vi "IFwTest.vi"() -> ()   [LabVIEW 2017]
uses:
  <vilib>/Platform/TimedLoop/XDataNode/timing_clust.ctl
  <vilib>/Platform/TimedLoop/XDataNode/nitl_modes.ctl
  <vilib>/Platform/TimedLoop/XDataNode/wakeup.ctl
  <instrlib>/_niInstr/Instruction Framework/v1/FPGA/Helper Classes/Single Address Space Collection/Single Address Space Collection.lvclass
  C:/Program Files (x86)/National Instruments/LabVIEW 2017/instr.lib/_niInstr/Instruction Framework/v1/FPGA/Interfaces/Address Space Collection/Address Space Collection.lvclass
  <instrlib>/_niInstr/FIFO Register Bus/v1/FPGA/niInstr FIFO Register Bus v1 FPGA.lvclass
  C:/Program Files (x86)/National Instruments/LabVIEW 2017/instr.lib/_niInstr/Instruction Framework/v1/FPGA/Interfaces/Instruction Producer/Instruction Producer.lvclass
  <vilib>/rvi/Emulation/niFpgaGetClockAttributes.vi
  <vilib>/rvi/Emulation/niFpgaSctlEmulationGetInTimedLoop.vi
  <vilib>/rvi/Emulation/niFpgaEmulationReportErrorSimple.vi
  <vilib>/rvi/Emulation/niFpgaCriticalErrorInLSC.vi
  <vilib>/rvi/DataTransferAndStorage/Container/Common/niFpgaContainerExecOnDevCompGetState.vi
  <vilib>/rvi/Emulation/niFpgaEmulationIsFPGAContextNoSignature.vi
  <vilib>/rvi/DataTransferAndStorage/Container/Common/niFpgaContainerGetUniqueNameForEmu.vi
  <vilib>/rvi/Memory/Memory_Emulation/niFpgaMemoryEmulationCacheClearOnFirstRun.vi
  <vilib>/rvi/Memory/Memory_Emulation/nirvimemoryEmulationManagerCache_MakeExclusive.vi
  <vilib>/rvi/Memory/Memory_Emulation/niFpgaMemoryEmulationValidateCache.vi
  <vilib>/rvi/Memory/Memory_Emulation/nirvimemoryEmulationManagerCache_InsertValue.vi
  <vilib>/Utility/error.llb/Clear Errors.vi
  <vilib>/rvi/Memory/Memory_Emulation/nirvimemoryEmulationManagerCache_ReleaseExclusive.vi
  <vilib>/rvi/Memory/Memory_Emulation/nirvimemoryEmulationManagerCache_GetValue.vi
  <vilib>/rvi/Memory/Memory_Emulation/nirvimemoryEmulationManagerCache_SetValue.vi
  <vilib>/rvi/Emulation/niFpgaProcessEmulError.vi
  <vilib>/Platform/TimedLoop/XDataNode/XDataNode.xnode
  <vilib>/rvi/DataTransferAndStorage/Container/XNode/niFpgaContainer.xnode
  <vilib>/rvi/DataTransferAndStorage/Register/Emulation/niFpgaRegisterEmulationRefIn.vi
  <instrlib>/_niInstr/Instruction Framework/v1/FPGA/Top Level Bus/Register Configuration/Register Configuration.lvclass
  <vilib>/Platform/TimedLoop/XDataNode/XDNodeRunTimeDep.lvlib
  AddressSpace.lvclass
panel:
  out "numOfInterleaves 2":u8
  out "rampRate 2":sgl
  out "manualInput 2":sgl
  out "perturbAmp 2":sgl
  out "perturbAngleInc 2":fxp<+/-,16,0>
  out "reset 2":bool
  out "state 2":T1(ring)
  out "gains 2":T2
  out "numInterleaves 2":u8
  out "enable 2":bool
  out "triangleInc 2":fxp<+,18,0>
  out "deadband 2":u16
  out "deadband":u16
  out "triangleInc":fxp<+,18,0>
  out "enable":bool
  out "numInterleaves":u8
  out "gains":T2
  out "state":T1(ring)
  out "reset":bool
  out "perturbAngleInc":fxp<+/-,16,0>
  out "perturbAmp":sgl
  out "manualInput":sgl
  out "rampRate":sgl
  out "numOfInterleaves":u8
  in  "fifo reg bus ctrl 0":u32
  out "fifo reg bus status 0":u32
  out "fifo reg bus data 0":u64
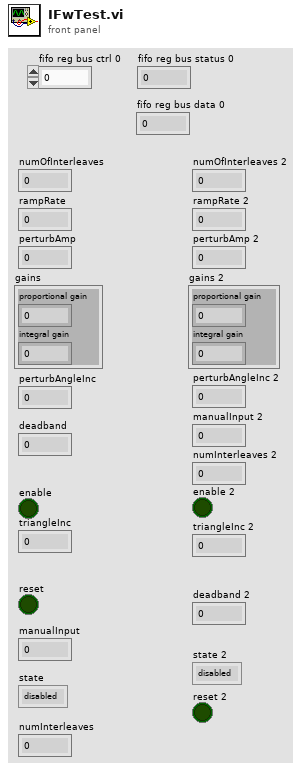
[diagram p1: front panel]
types:
  T1 = enum16{"disabled", "manual", "normal", "perturb"}
  T2 = cluster{"proportional gain":sgl, "integral gain":sgl}
  T3 = typedef "XDNodeRunTimeDep.lvlib/timing_clust.ctl" = cluster{"Expected End [f-1]":u64, "Actual End [f-1]":u64, "Finished Late? [f-1]":bool, "Expected End [i-1]":u64, "Actual End [i-1]":u64, "Finished Late? [i-1]":bool, "Expected Start [i]":u64, "Actual Start [i]":u64, "Expected Start [f]":u64, "Actual Start [f]":u64, "Source Name":string, "Structure Name":string, "Period":i64, "Deadline":i64, "Offset":i64, "Start":i64, "Priority":i32, "Timeout":i32, "Mode":T4, "Wakeup Reason":T5, "Error":errorcluster, "Source Type":string, "Secondary Source Type":string, "Global End Time":u64, "Global Start Time":u64, "Frame Duration":u64, "Iteration Duration":u64, "Assigned CPU":i32, "I/O Scan Engine Mode":u32}
  T4 = typedef "XDNodeRunTimeDep.lvlib/nitl_modes.ctl" = enum32{"No Change", "Process missed periods, maintain original phase", "Discard missed periods, maintain original phase", "Process missed periods, ignore original phase", "Discard missed periods, ignore original phase"}
  T5 = typedef "XDNodeRunTimeDep.lvlib/wakeup.ctl" = enum32{"Normal", "Aborted", "Asynchronous wakeup", "Timing source error", "Timed loop error", "Timeout"}
  T6 = typedef "BuckBoost.lvlib/contSettings.ctl" = cluster{"numberOfInterleaves":refnum<k21>, "rampRate":refnum<k21>, "manualInput":refnum<k21>, "perturbAmp":refnum<k21>, "perturbAngleInc":refnum<k21>, "reset":refnum<k21>, "state":refnum<k21>, "gains":refnum<k21>}
  T7 = typedef "BuckBoost.lvlib/modRegisters.ctl" = cluster{"numberOfInterleaves":refnum<k21>, "Enable":refnum<k21>, "triangleInc":refnum<k21>, "Deadband":refnum<k21>}
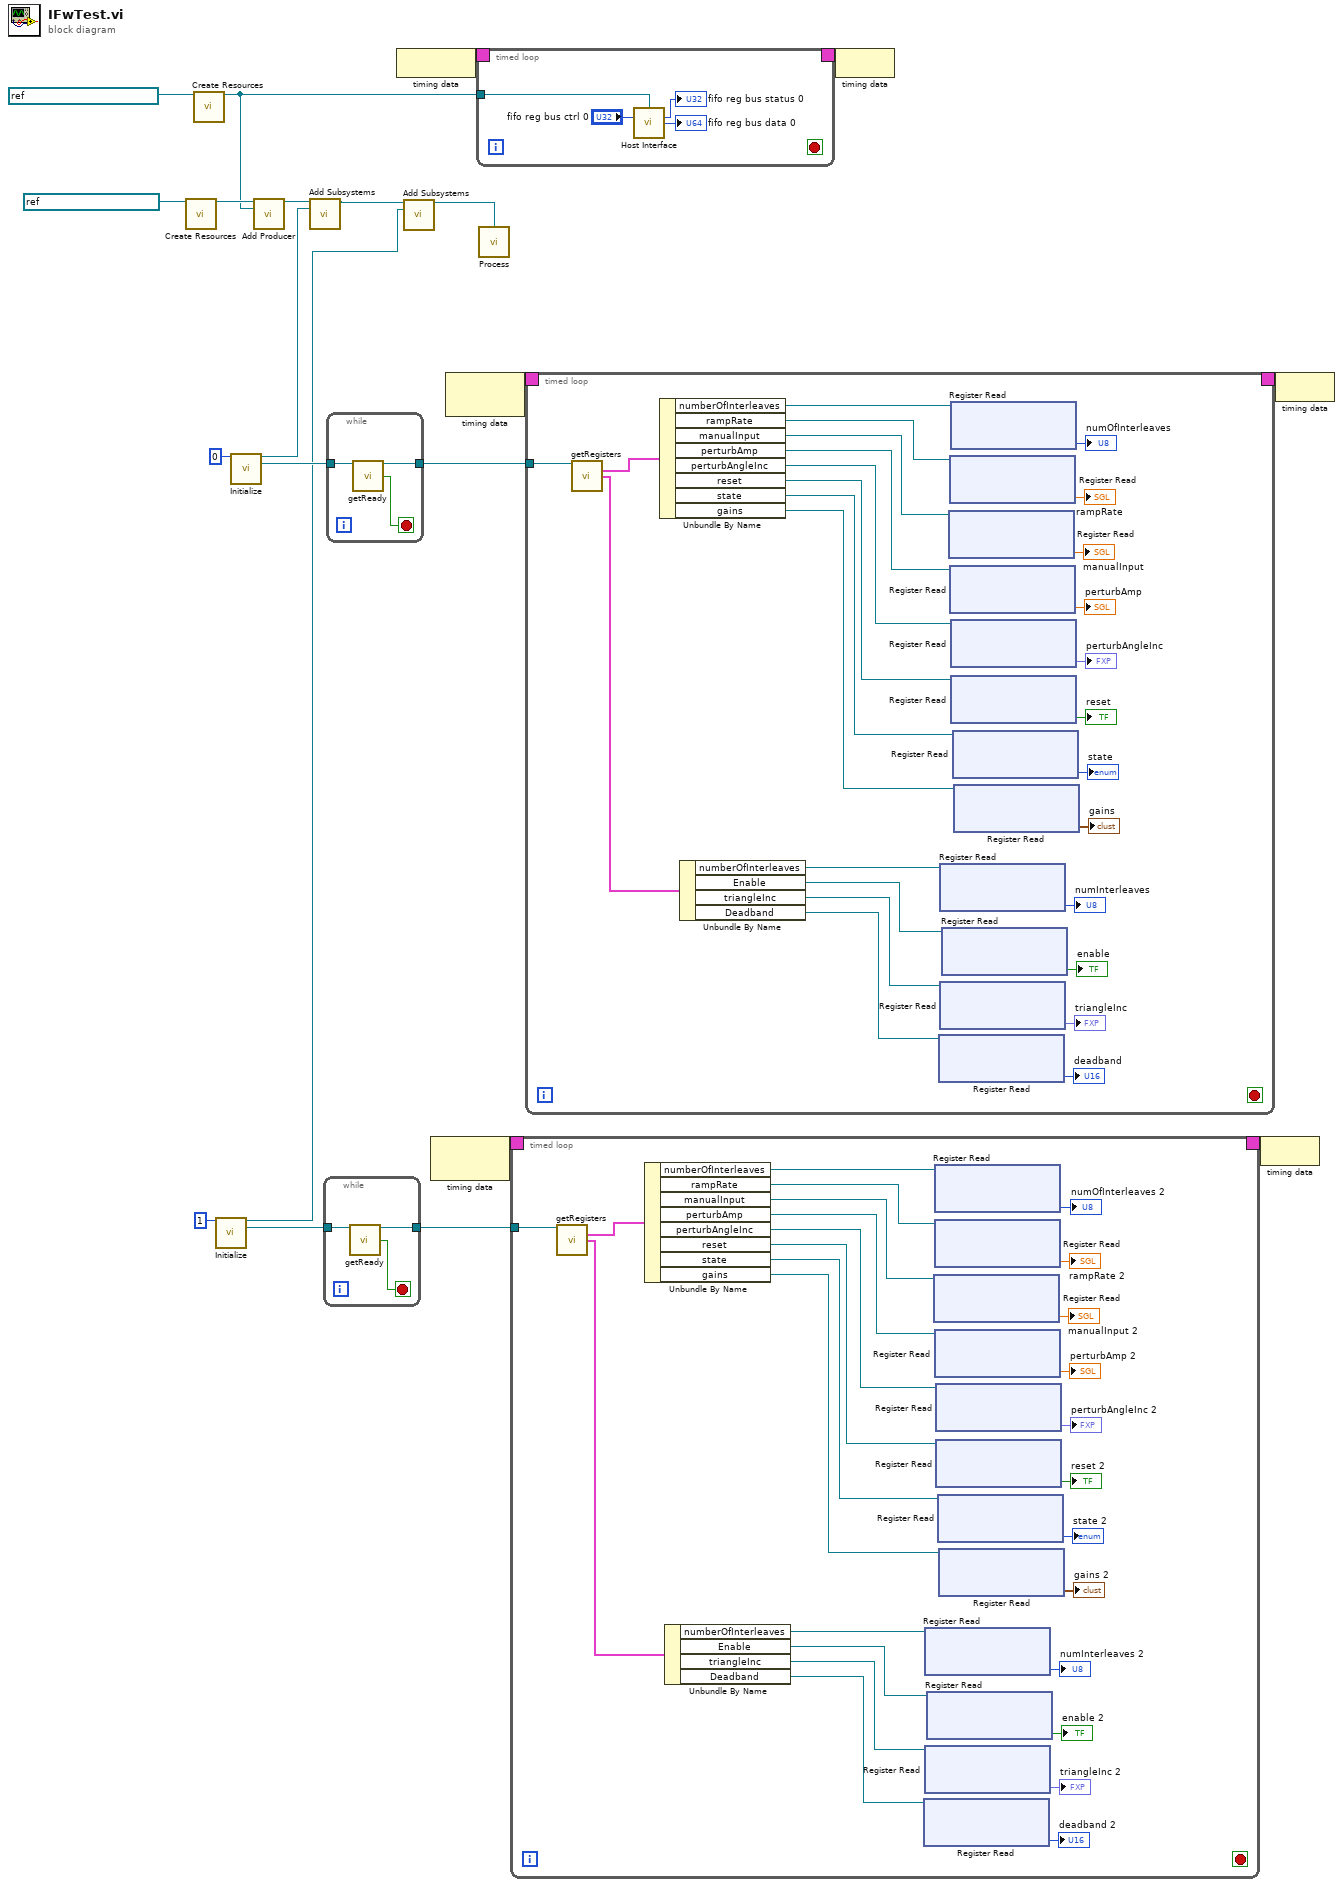
[diagram p0: block diagram]
diagram:
  n1 = call <instrlib>:"Create Resources.vi"("register clock"=refnum<k21> "40 MHz Onboard Clock") -> ("register configuration"=w19:refnum<class "Register Configuration.lvclass">)  [unwired: 14 in]
  n2 = call <instrlib>:"Create Resources.vi"("instruction fifo"=refnum<k21> "reg.host instruction fifo 0") -> ("fifo register bus"=w15:refnum<class "niInstr FIFO Register Bus v1 FPGA.lvclass">)  [unwired: 14 in]
  n3 = call "Initialize.vi"("instance"=u8 1) -> ("subsystem"=w6:refnum<class "Single Address Space Collection.lvclass">, "AddressSpace"=w1:refnum<class "AddressSpace.lvclass">)  [unwired: 13 in]
  n4 = call "Initialize.vi"("instance"=u8 0) -> ("subsystem"=w11:refnum<class "Single Address Space Collection.lvclass">, "AddressSpace"=w12:refnum<class "AddressSpace.lvclass">)  [unwired: 13 in]
  n5 = call <instrlib>:"Add Producer.vi"("register configuration in"=w19, "instruction producer"=w15) -> ("register configuration out"=w17:refnum<class "Register Configuration.lvclass">)  [unwired: 13 in]
  n6 = call <instrlib>:"Add Subsystems.vi"("register configuration in"=w17, "subsystems"=w11) -> ("register configuration out"=w13:refnum<class "Register Configuration.lvclass">)  [unwired: 13 in]
  n7 = while {
    tunnel: w1 -> [w24]
    tunnel: [w23] -> w3
    stop <- w22 stop-if-true
    n8 = call "getReady.vi"("AddressSpace in"=w24) -> ("AddressSpace out"=w23:refnum<class "AddressSpace.lvclass">, "ready"=w22:bool)  [unwired: 13 in]
  }
  n9 = while {
    tunnel: w12 -> [w27]
    tunnel: [w26] -> w9
    stop <- w25 stop-if-true
    n10 = call "getReady.vi"("AddressSpace in"=w27) -> ("AddressSpace out"=w26:refnum<class "AddressSpace.lvclass">, "ready"=w25:bool)  [unwired: 13 in]
  }
  n11 = node-c288() -> (w21:T3)
  n12 = call <instrlib>:"Add Subsystems.vi"("register configuration in"=w13, "subsystems"=w6) -> ("register configuration out"=w14:refnum<class "Register Configuration.lvclass">)  [unwired: 13 in]
  n13 = node-c288() -> (w5:T3)  [unwired: 1 in]
  n14 = node-c288() -> (w8:T3)  [unwired: 1 in]
  n15 = timed-loop {
    timing: w21 -> [_]
    timing-out: [_] -> w20
    tunnel: w15 -> [w31]
    stop <- _ stop-if-true
    n16 = call <instrlib>:"Host Interface.vi"("fifo register bus"=w31, "fifo reg bus ctrl 0"="fifo reg bus ctrl 0") -> ("fifo reg bus status 0"=→"fifo reg bus status 0":u32, "fifo reg bus data 0"=→"fifo reg bus data 0":u64)  [unwired: 12 in]
  }
  n17 = call <instrlib>:"Process.vi"("register configuration"=w14) -> ()  [unwired: 15 in]
  n18 = timed-loop {
    timing: w5 -> [_]
    timing-out: [_] -> w4
    tunnel: w3 -> [w60]
    stop <- _ stop-if-true
    n19 = call "getRegisters.vi"("AddressSpace in"=w60) -> ("settingsReg"=w59:T6, "modRegisters"=w58:T7)  [unwired: 12 in, 1 out]
    n20 = Unbundle By Name(w59) -> ("numberOfInterleaves"=w35:refnum<k21>, "rampRate"=w57:refnum<k21>, "manualInput"=w56:refnum<k21>, "perturbAmp"=w55:refnum<k21>, "perturbAngleInc"=w54:refnum<k21>, "reset"=w53:refnum<k21>, "state"=w52:refnum<k21>, "gains"=w51:refnum<k21>)
    n21 = Unbundle By Name(w58) -> ("numberOfInterleaves"=w50:refnum<k21>, "Enable"=w49:refnum<k21>, "triangleInc"=w48:refnum<k21>, "Deadband"=w47:refnum<k21>)
    n22 = xnode ("Register Read")("Register In"=w47) -> ("Data"=→"deadband 2":u16)  [unwired: 1 out]
    n23 = xnode ("Register Read")("Register In"=w50) -> ("Data"=→"numInterleaves 2":u8)  [unwired: 1 out]
    n24 = xnode ("Register Read")("Register In"=w48) -> ("Data"=→"triangleInc 2":fxp<+,18,0>)  [unwired: 1 out]
    n25 = xnode ("Register Read")("Register In"=w49) -> ("Data"=→"enable 2":bool)  [unwired: 1 out]
    n26 = xnode ("Register Read")("Register In"=w56) -> ("Data"=→"manualInput 2":sgl)  [unwired: 1 out]
    n27 = xnode ("Register Read")("Register In"=w35) -> ("Data"=→"numOfInterleaves 2":u8)  [unwired: 1 out]
    n28 = xnode ("Register Read")("Register In"=w57) -> ("Data"=→"rampRate 2":sgl)  [unwired: 1 out]
    n29 = xnode ("Register Read")("Register In"=w55) -> ("Data"=→"perturbAmp 2":sgl)  [unwired: 1 out]
    n30 = xnode ("Register Read")("Register In"=w54) -> ("Data"=→"perturbAngleInc 2":fxp<+/-,16,0>)  [unwired: 1 out]
    n31 = xnode ("Register Read")("Register In"=w53) -> ("Data"=→"reset 2":bool)  [unwired: 1 out]
    n32 = xnode ("Register Read")("Register In"=w52) -> ("Data"=→"state 2":T1)  [unwired: 1 out]
    n33 = xnode ("Register Read")("Register In"=w51) -> ("Data"=→"gains 2":T2)  [unwired: 1 out]
  }
  n34 = timed-loop {
    timing: w8 -> [_]
    timing-out: [_] -> w7
    tunnel: w9 -> [w89]
    stop <- _ stop-if-true
    n35 = call "getRegisters.vi"("AddressSpace in"=w89) -> ("settingsReg"=w88:T6, "modRegisters"=w87:T7)  [unwired: 12 in, 1 out]
    n36 = Unbundle By Name(w88) -> ("numberOfInterleaves"=w86:refnum<k21>, "rampRate"=w85:refnum<k21>, "manualInput"=w84:refnum<k21>, "perturbAmp"=w83:refnum<k21>, "perturbAngleInc"=w82:refnum<k21>, "reset"=w81:refnum<k21>, "state"=w80:refnum<k21>, "gains"=w79:refnum<k21>)
    n37 = Unbundle By Name(w87) -> ("numberOfInterleaves"=w78:refnum<k21>, "Enable"=w77:refnum<k21>, "triangleInc"=w76:refnum<k21>, "Deadband"=w75:refnum<k21>)
    n38 = xnode ("Register Read")("Register In"=w75) -> ("Data"=→"deadband":u16)  [unwired: 1 out]
    n39 = xnode ("Register Read")("Register In"=w78) -> ("Data"=→"numInterleaves":u8)  [unwired: 1 out]
    n40 = xnode ("Register Read")("Register In"=w76) -> ("Data"=→"triangleInc":fxp<+,18,0>)  [unwired: 1 out]
    n41 = xnode ("Register Read")("Register In"=w77) -> ("Data"=→"enable":bool)  [unwired: 1 out]
    n42 = xnode ("Register Read")("Register In"=w84) -> ("Data"=→"manualInput":sgl)  [unwired: 1 out]
    n43 = xnode ("Register Read")("Register In"=w85) -> ("Data"=→"rampRate":sgl)  [unwired: 1 out]
    n44 = xnode ("Register Read")("Register In"=w83) -> ("Data"=→"perturbAmp":sgl)  [unwired: 1 out]
    n45 = xnode ("Register Read")("Register In"=w86) -> ("Data"=→"numOfInterleaves":u8)  [unwired: 1 out]
    n46 = xnode ("Register Read")("Register In"=w82) -> ("Data"=→"perturbAngleInc":fxp<+/-,16,0>)  [unwired: 1 out]
    n47 = xnode ("Register Read")("Register In"=w81) -> ("Data"=→"reset":bool)  [unwired: 1 out]
    n48 = xnode ("Register Read")("Register In"=w80) -> ("Data"=→"state":T1)  [unwired: 1 out]
    n49 = xnode ("Register Read")("Register In"=w79) -> ("Data"=→"gains":T2)  [unwired: 1 out]
  }
  n50 = node-c288(w20) -> ()
  n51 = node-c288(w4) -> ()
  n52 = node-c288(w7) -> ()
